vi "Create Stream.vi"(8 "error in (no error)":errorcluster, 10 "IP":string="//localhost", 11 "Channel in":refnum<class "Channel.lvclass">) -> (0 "error out":errorcluster, 3 "Channel out":refnum<class "Channel.lvclass">)   [LabVIEW 2018, in "Channel.lvclass"]
uses:
  Channel.lvclass
  Stream/Stream.lvclass
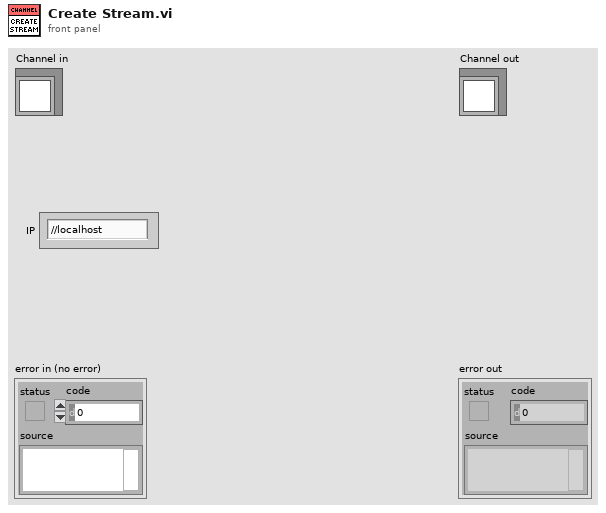
[diagram p1: front panel]
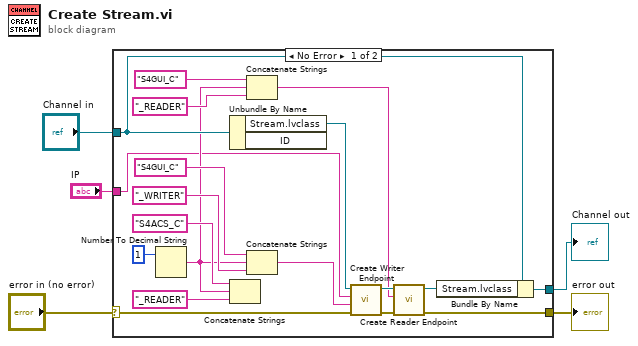
[diagram p0: block diagram]
diagram:
  n1 = case shown="No Error" "error in (no error)" {
    selector: "error in (no error)" -> [w11 w26]
    tunnel: [w8 w26] -> w3
    tunnel: [w23 w25] -> w2
    tunnel: "Channel in" -> [w24 w25]
    tunnel: "IP" -> [w13 _]
    frame No Error {
      n2 = Number To Decimal String(number=1) -> (decimal integer string=w16:string)  [unwired: 1 in]
      n3 = Unbundle By Name(w24) -> ("Stream.lvclass"=w14:refnum<class "Stream.lvclass">)  [unwired: 1 out]
      n4 = Concatenate Strings("S4ACS_C" ("reader name"), w16, "_READER" ("reader name")) -> ()  [unwired: 1 out]
      n5 = Concatenate Strings("S4GUI_C" ("reader name"), w16, "_READER" ("reader name")) -> (w7:string)
      n6 = Concatenate Strings("S4GUI_C", w16, "_WRITER") -> (w12:string)
      n7 = call "Create Writer Endpoint.vi"("error in (no error)"=w11, "reader name"=w12, "IP"=w13, "Stream in"=w14) -> ("error out"=w9:errorcluster, "Stream out"=w10:refnum<class "Stream.lvclass">)  [unwired: 6 in]
      n8 = call "Create Reader Endpoint.vi"("error in (no error)"=w9, "reader name"=w7, "Stream in"=w10) -> ("error out"=w8:errorcluster, "Stream out"=w6:refnum<class "Stream.lvclass">)  [unwired: 7 in]
      n9 = Bundle By Name(cluster=w24, "Stream.lvclass"=w6) -> (w23:refnum<class "Channel.lvclass">)
    }
    frame Error {
    }
  }
  "error out" <- w3
  "Channel out" <- w2
